vi "SyncopationCalcExample.vi"() -> ()   [LabVIEW 2016]
panel:
  out "dutyArray":u16[](array[numeric]) format="%016b"
  in  "Loops":i32
  in  "firstDuty":u16=257 format="%016b"
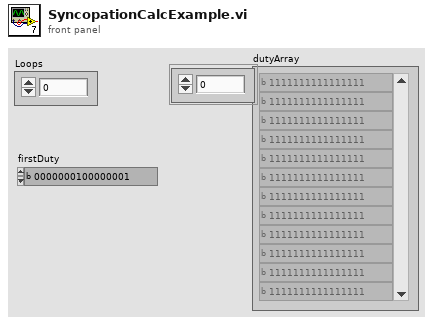
[diagram p1: front panel]
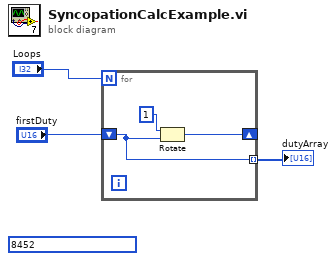
[diagram p0: block diagram]
diagram:
  (unwired) u16 8452 ("Duty")
  n1 = for {
    N: "Loops" -> [_]
    shift-right: [w5] -> _
    shift-left: "firstDuty" -> [w6]
    tunnel: [w6] -> w1 mode=indexing
    n2 = Rotate(1:w6, 2:i16 1 ("y")) -> (0:w5:u16)
  }
  "dutyArray" <- w1
